vi "LogicTrain-Sample-05-01.vi"() -> ()   [LabVIEW 2020]
uses:
  <vilib>/Rock Robotics/WPI/ThirdParty/JAS_Junk/TrajLib/Trajectory_Library.lvlib
panel:
  in  "Capture Cube":bool
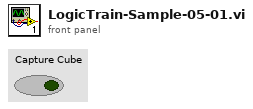
[diagram p1: front panel]
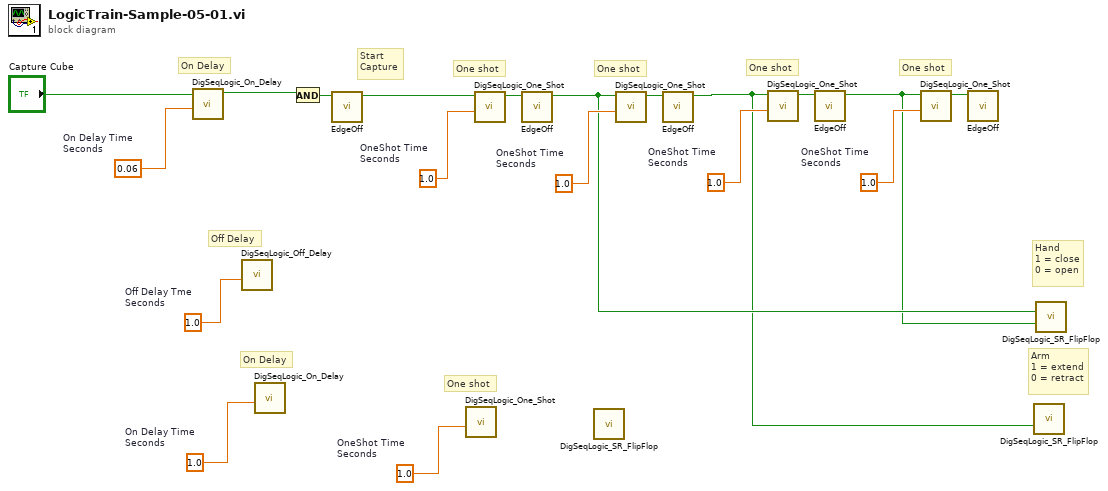
[diagram p0: block diagram]
diagram:
  w5 = 1.0  # OneShot Time Seconds
  w7 = 1.0  # OneShot Time Seconds
  w9 = 1.0  # OneShot Time Seconds
  w13 = 1.0  # OneShot Time Seconds
  w16 = 0.06  # On Delay Time Seconds
  w17 = 1.0  # OneShot Time Seconds
  w18 = 1.0  # On Delay Time Seconds
  w19 = 1.0  # Off Delay Tme Seconds
  # "Arm\n1 = extend\n0 = retract"
  # "Hand\n1 = close\n0 = open"
  # "One shot"
  # "One shot"
  # "One shot"
  # "Start\nCapture"
  # "One shot"
  # "On Delay"
  # "One shot"
  # "On Delay"
  # "Off Delay"
  n1 = call <vilib>:"DigSeqLogic_On_Delay.vi"("Delay"=w16, "Input"="Capture Cube") -> ("Output"=w14:bool)  [unwired: 8 in, 1 out]
  n2 = call <vilib>:"DigSeqLogic_Off_Delay.vi"("Delay"=w19) -> ()  [unwired: 9 in, 2 out]
  n3 = call <vilib>:"DigSeqLogic_On_Delay.vi"("Delay"=w18) -> ()  [unwired: 9 in, 2 out]
  n4 = And(x=w14) -> (x .and. y?=w12:bool)  [unwired: 1 in]
  n5 = call "EdgeOff.vi"("Input"=w12) -> ("Edge Off"=w11:bool)  [unwired: 10 in]
  n6 = call <vilib>:"DigSeqLogic_One_Shot.vi"("OneShot"=w17) -> ()  [unwired: 9 in, 2 out]
  n7 = call <vilib>:"DigSeqLogic_One_Shot.vi"("OneShot"=w13, "Input"=w11) -> ("Output"=w10:bool)  [unwired: 8 in, 1 out]
  n8 = call "EdgeOff.vi"("Input"=w10) -> ("Edge Off"=w3:bool)  [unwired: 10 in]
  n9 = call <vilib>:"DigSeqLogic_SR_FlipFlop.vi"() -> ()  [unwired: 14 in, 2 out]
  n10 = call <vilib>:"DigSeqLogic_One_Shot.vi"("OneShot"=w9, "Input"=w3) -> ("Output"=w8:bool)  [unwired: 8 in, 1 out]
  n11 = call "EdgeOff.vi"("Input"=w8) -> ("Edge Off"=w2:bool)  [unwired: 10 in]
  n12 = call <vilib>:"DigSeqLogic_One_Shot.vi"("OneShot"=w7, "Input"=w2) -> ("Output"=w6:bool)  [unwired: 8 in, 1 out]
  n13 = call "EdgeOff.vi"("Input"=w6) -> ("Edge Off"=w1:bool)  [unwired: 10 in]
  n14 = call <vilib>:"DigSeqLogic_One_Shot.vi"("OneShot"=w5, "Input"=w1) -> ("Output"=w4:bool)  [unwired: 8 in, 1 out]
  n15 = call "EdgeOff.vi"("Input"=w4) -> ()  [unwired: 10 in, 1 out]
  n16 = call <vilib>:"DigSeqLogic_SR_FlipFlop.vi"("Reset"=w2) -> ()  [unwired: 13 in, 2 out]
  n17 = call <vilib>:"DigSeqLogic_SR_FlipFlop.vi"("Set"=w3, "Reset"=w1) -> ()  [unwired: 12 in, 2 out]
